vi "Check for Input.vi"(8 "error in (no error)":errorcluster, 9 "Control Refs":refnum<vi>[](array[refnum]), 10 "Mouse Ref":refnum<k1>, 11 "Mouse Action in":refnum<class "Mouse Action.lvclass">) -> (0 "error out":errorcluster, 3 "Mouse Action out":refnum<class "Mouse Action.lvclass">)   [LabVIEW 2020, in "MacroAssert.lvlib" / "Mouse Action.lvclass"]
uses:
  Mouse Action.lvclass
  Mouse Action.lvclass/Mouse Action.ctl
  <vilib>/Utility/inputDevices.llb/mouseAcquire.vi
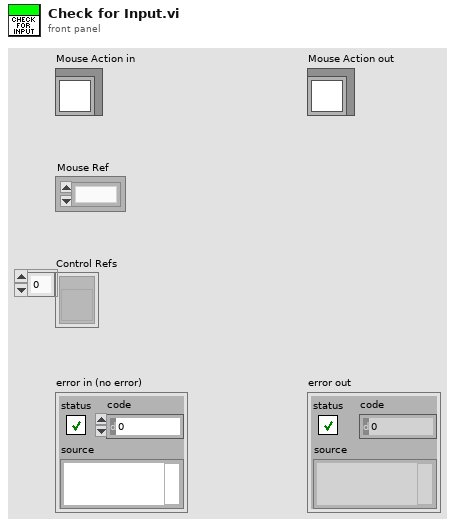
[diagram p1: front panel]
types:
  T1 = cluster{"Horizontal":i32, "Vertical":i32, "Scrolling":i32}
  T2 = cluster{"button 1":bool, "button 2":bool, "button 3":bool, "button 4":bool}
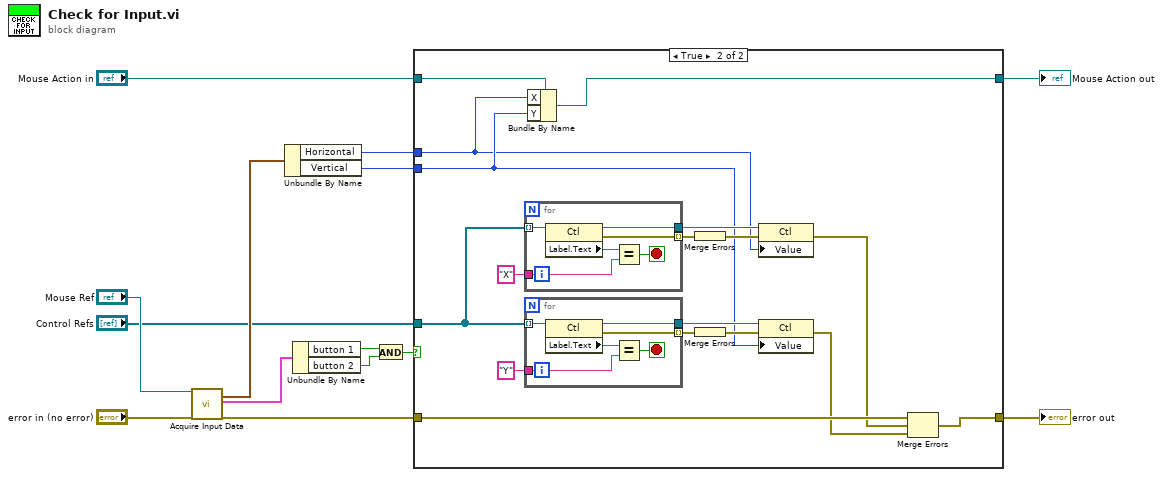
[diagram p0: block diagram]
diagram:
  n1 = call-poly <vilib>:"Acquire Input Data.vi"("device ID"="Mouse Ref", "error in (no error)"="error in (no error)") -> ("axis info"=w10:T1, "button info"=w11:T2, "error out"=w2:errorcluster)  [unwired: 14 in, 1 out]
  n2 = Unbundle By Name(w10) -> ("Horizontal"=w6:i32, "Vertical"=w5:i32)
  n3 = Unbundle By Name(w11) -> ("button 1"=w8:bool, "button 2"=w9:bool)
  n4 = And(x=w8, y=w9) -> (x .and. y?=w7:bool)
  n5 = case shown="True" w7 {
    tunnel: w6 -> [_ w17]
    tunnel: w5 -> [_ w18]
    tunnel: "Mouse Action in" -> [w16 w33]
    tunnel: [w16 w32] -> w4
    tunnel: "Control Refs" -> [_ w21]
    tunnel: w2 -> [w15 w27]
    tunnel: [w15 w26] -> w1
    frame False {
    }
    frame True {
      n6 = for {
        tunnel: w21 -> [w45] mode=indexing
        tunnel: [w44] -> w31
        tunnel: "X" -> [w41]
        tunnel: [w40] -> w29 mode=indexing
        stop <- w42 stop-if-true
        n7 = property class="Ctl"(reference=w45) -> (reference out=w44:refnum<vi>, error out=w40:errorcluster, "Label.Text"=w43:string)  [unwired: 1 in]
        n8 = Equal?(x=w43, y=w41) -> (x = y?=w42:bool)
      }
      n9 = for {
        tunnel: w21 -> [w39] mode=indexing
        tunnel: [w38] -> w22
        tunnel: "Y" -> [w35]
        tunnel: [w34] -> w24 mode=indexing
        stop <- w36 stop-if-true
        n10 = property class="Ctl"(reference=w39) -> (reference out=w38:refnum<vi>, error out=w34:errorcluster, "Label.Text"=w37:string)  [unwired: 1 in]
        n11 = Equal?(x=w37, y=w35) -> (x = y?=w36:bool)
      }
      n12 = Bundle By Name(cluster=w33, "X"=w17, "Y"=w18) -> (w32:refnum<class "Mouse Action.lvclass">)
      n13 = Merge Errors(w29) -> (w28:errorcluster)
      n14 = Merge Errors(w24) -> (w25:errorcluster)
      n15 = property class="Ctl"(reference=w31, error in=w28, "Value"=w17) -> (error out=w19:errorcluster)  [unwired: 1 out]
      n16 = property class="Ctl"(reference=w22, error in=w25, "Value"=w18) -> (error out=w20:errorcluster)  [unwired: 1 out]
      n17 = Merge Errors(w27, w19, w20) -> (w26:errorcluster)
    }
  }
  "error out" <- w1
  "Mouse Action out" <- w4
